vi "test-math-utils.vi"(8 "error in (no error)":errorcluster) -> (0 "error out":errorcluster, 3 "ALL TESTS PASSED":bool)   [LabVIEW 2019]
uses:
  <vilib>/Rock Robotics/WPI/ThirdParty/JAS_Junk/TrajLib/Trajectory_Library.lvlib
panel:
  out "Test 40":bool
  out "Test 39":bool
  out "Test 38":bool
  out "Test 37":bool
  out "Test 36":bool
  out "Test 35":bool
  out "Test 34":bool
  out "Test 33":bool
  out "Test 32":bool
  out "Test 31":bool
  out "Test 30":bool
  out "Test 29":bool
  out "Test 28":bool
  out "Test 27":bool
  out "Test 26":bool
  out "Test 25":bool
  out "mod 24":dbl
  out "Test 24":bool
  out "mod 23":dbl
  out "Test 23":bool
  out "mod 22":dbl
  out "Test 22":bool
  out "mod 21":dbl
  out "Test 21":bool
  out "mod 20":dbl
  out "Test 20":bool
  out "mod 19":dbl
  out "Test 19":bool
  out "mod 18":dbl
  out "mod 17":dbl
  out "mod 16":dbl
  out "Test 18":bool
  out "Test 17":bool
  out "Test 16":bool
  out "Test 15":bool
  out "Test 14":bool
  out "Test 13":bool
  out "Test 12":bool
  out "Test 11":bool
  out "Test 10":bool
  out "Test 9":bool
  out "Test 8":bool
  out "Test 7":bool
  out "Test 6":bool
  out "Test 5":bool
  out "Test 4":bool
  out "Test 3":bool
  out "Test 2":bool
  out "Test 1":bool
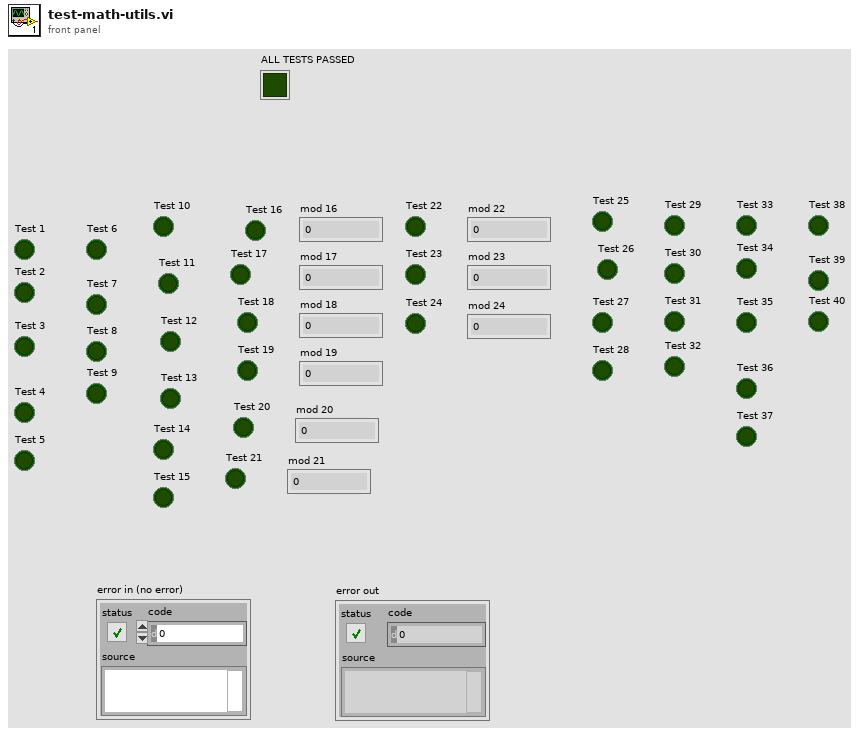
[diagram p1: front panel]
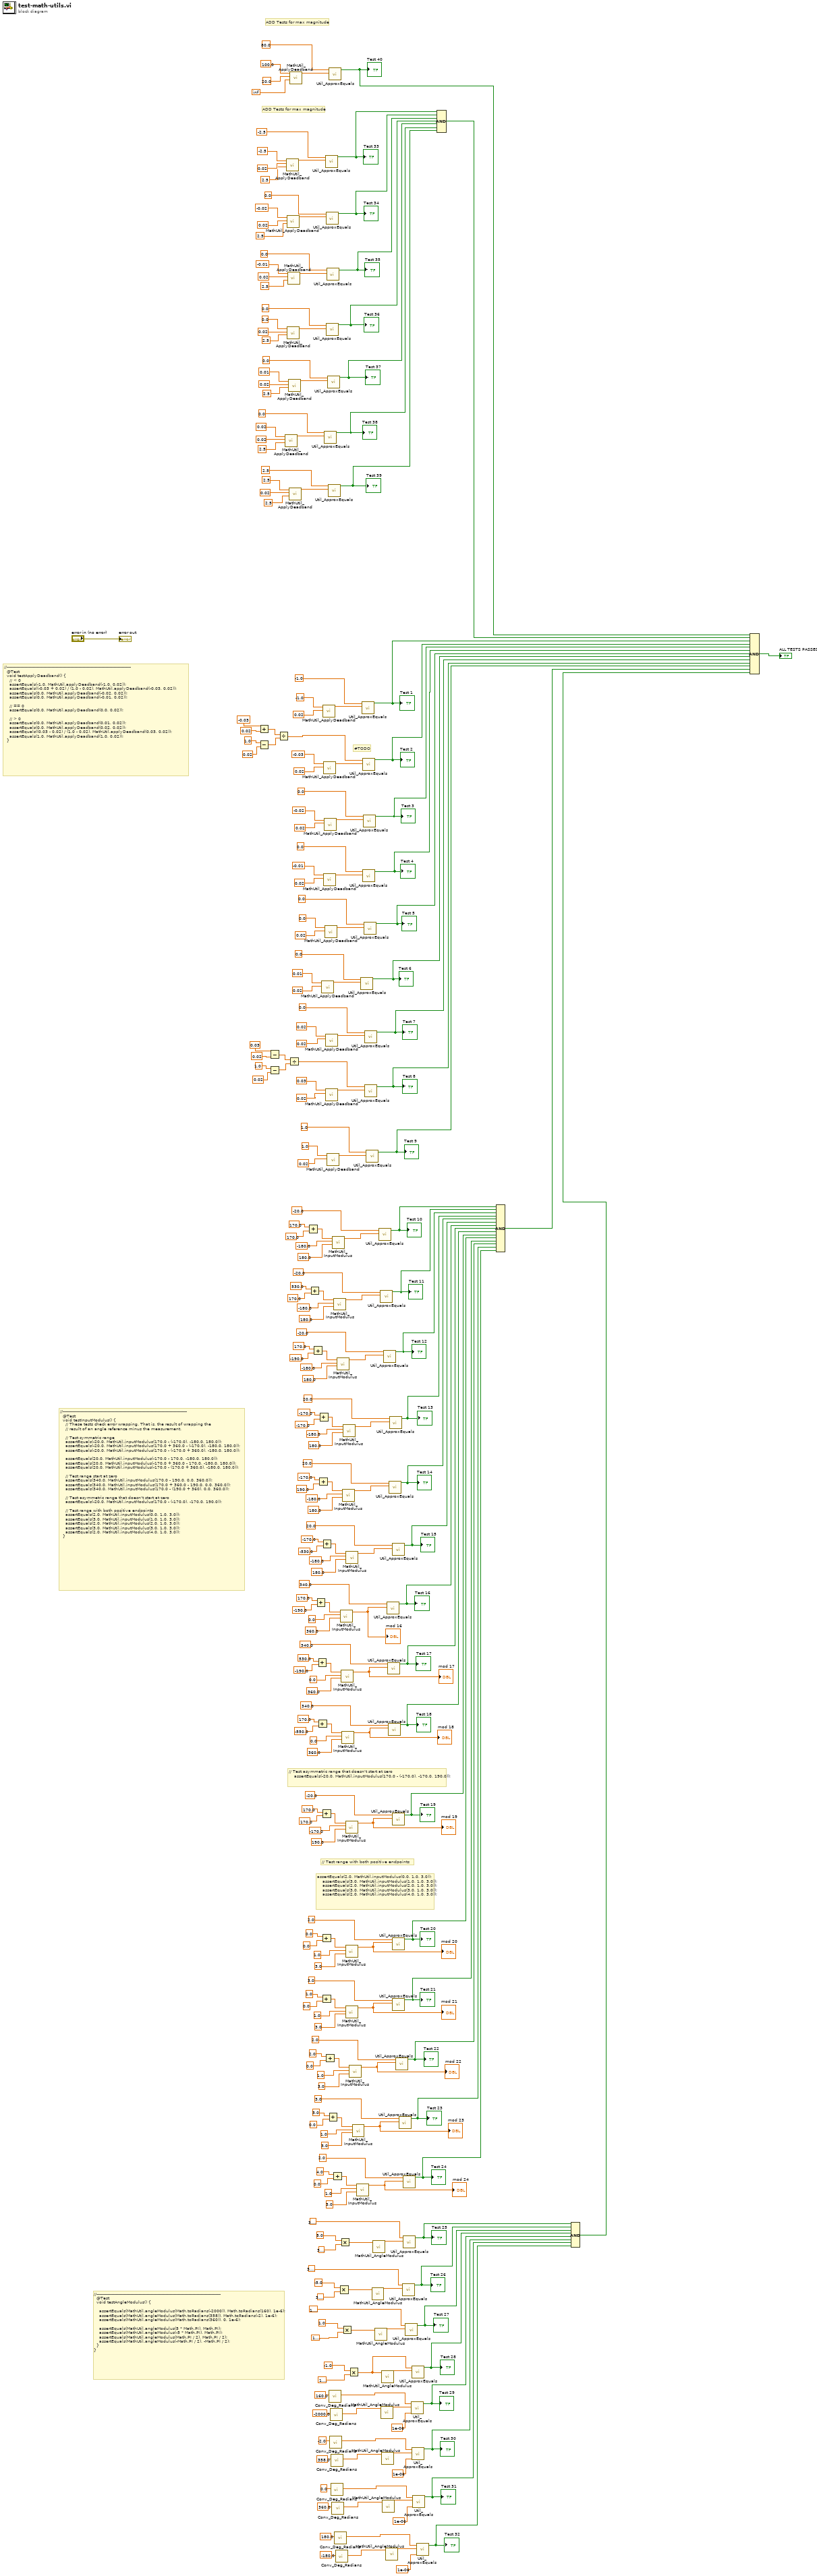
[diagram p0: block diagram]
diagram:
  # "ADD Tests for max magnitude"
  # "ADD Tests for max magnitude"
  # "assertEquals(2.0, MathUtil.inputModulus(0.0, 1.0, 3.0));\n    assertEquals(3.0, MathUtil.inputModulus(1.0, 1.0, 3.0));\n    assertEquals(2.0, MathUtil.inputModulus(2.0, 1.0, 3.0));\n    assertEquals(3.0, MathUtil.inputModulus(3.0, 1.0, 3.0));\n    assertEquals(2.0, MathUtil.inputModulus(4.0, 1.0, 3.0));"
  # "// Test range with both positive endpoints"
  # "// Test asymmetric range that doesn't start at zero\n    assertEquals(-20.0, MathUtil.inputModulus(170.0 - (-170.0), -170.0, 190.0));"
  # "#TODO"
  # "//--------------------------------------------------------------------------------------------\n  @Test\n  void testInputModulus() {\n    // These tests check error wrapping. That is, the result of wrapping the\n    // result of an angle reference minus the measurement.\n\n    // Test symmetric range\n    assertEquals(-20.0, MathUtil.inputModulus(170.0 - (-170.0), -180.0, 180.0));\n    assertEquals(-20.0, MathUtil.inputModulus(170.0 + 360.0 - (-170.0), -180.0, 180.0));\n    assertEquals(-20.0, MathUtil.inputModulus(170.0 - (-170.0 + 360.0), -180.0, 180.0));\n\n    assertEquals(20.0, MathUtil.inputModulus(-170.0 - 170.0, -180.0, 180.0));\n    assertEquals(20.0, MathUtil.inputModulus(-170.0 + 360.0 - 170.0, -180.0, 180.0));\n    assertEquals(20.0, MathUtil.inputModulus(-170.0 - (170.0 + 360.0), -180.0, 180.0));\n\n    // Test range start at zero\n    assertEquals(340.0, MathUtil.inputModulus(170.0 - 190.0, 0.0, 360.0));\n    assertEquals(340.0, MathUtil.inputModulus(170.0 + 360.0 - 190.0, 0.0, 360.0));\n    assertEquals(340.0, MathUtil.inputModulus(170.0 - (190.0 + 360), 0.0, 360.0));\n\n    // Test asymmetric range that doesn't start at zero\n    assertEquals(-20.0, MathUtil.inputModulus(170.0 - (-170.0), -170.0, 190.0));\n\n    // Test range with both positive endpoints\n    assertEquals(2.0, MathUtil.inputModulus(0.0, 1.0, 3.0));\n    assertEquals(3.0, MathUtil.inputModulus(1.0, 1.0, 3.0));\n    assertEquals(2.0, MathUtil.inputModulus(2.0, 1.0, 3.0));\n    assertEquals(3.0, MathUtil.inputModulus(3.0, 1.0, 3.0));\n    assertEquals(2.0, MathUtil.inputModulus(4.0, 1.0, 3.0));\n  }"
  # "//--------------------------------------------------------------------------------------------\n  @Test\n  void testApplyDeadband() {\n    // < 0\n    assertEquals(-1.0, MathUtil.applyDeadband(-1.0, 0.02));\n    assertEquals((-0.03 + 0.02) / (1.0 - 0.02), MathUtil.applyDeadband(-0.03, 0.02));\n    assertEquals(0.0, MathUtil.applyDeadband(-0.02, 0.02));\n    assertEquals(0.0, MathUtil.applyDeadband(-0.01, 0.02));\n\n    // == 0\n    assertEquals(0.0, MathUtil.applyDeadband(0.0, 0.02));\n\n    // > 0\n    assertEquals(0.0, MathUtil.applyDeadband(0.01, 0.02));\n    assertEquals(0.0, MathUtil.applyDeadband(0.02, 0.02));\n    assertEquals((0.03 - 0.02) / (1.0 - 0.02), MathUtil.applyDeadband(0.03, 0.02));\n    assertEquals(1.0, MathUtil.applyDeadband(1.0, 0.02));\n  }"
  # "//--------------------------------------------------------------------------------------------\n  @Test\n  void testAngleModulus() {\n\n    assertEquals(MathUtil.angleModulus(Math.toRadians(-2000)), Math.toRadians(160), 1e-6);\n    assertEquals(MathUtil.angleModulus(Math.toRadians(358)), Math.toRadians(-2), 1e-6);\n    assertEquals(MathUtil.angleModulus(Math.toRadians(360)), 0, 1e-6);\n\n    assertEquals(MathUtil.angleModulus(5 * Math.PI), Math.PI);\n    assertEquals(MathUtil.angleModulus(-5 * Math.PI), Math.PI);\n    assertEquals(MathUtil.angleModulus(Math.PI / 2), Math.PI / 2);\n    assertEquals(MathUtil.angleModulus(-Math.PI / 2), -Math.PI / 2);\n  }\n}"
  n1 = Add(x=-0.03, y=0.02) -> (x+y=w245:dbl)
  n2 = Subtract(x=1.0, y=0.02) -> (x-y=w244:dbl)
  n3 = Subtract(x=0.03, y=0.02) -> (x-y=w238:dbl)
  n4 = Subtract(x=1.0, y=0.02) -> (x-y=w237:dbl)
  n5 = Divide(x=w245, y=w244) -> (x/y=w239:dbl)
  n6 = call <vilib>:"MathUtil_ApplyDeadband.vi"("Max Magnitude"=2.5, "Deadband"=0.02, "Value"=0.02) -> ("Result"=w34:dbl)  [unwired: 8 in]
  n7 = call <vilib>:"MathUtil_ApplyDeadband.vi"("Max Magnitude"=2.5, "Deadband"=0.02, "Value"=-2.5) -> ("Result"=w48:dbl)  [unwired: 8 in]
  n8 = call <vilib>:"MathUtil_ApplyDeadband.vi"("Max Magnitude"=2.5, "Deadband"=0.02, "Value"=-0.02) -> ("Result"=w46:dbl)  [unwired: 8 in]
  n9 = call <vilib>:"MathUtil_ApplyDeadband.vi"("Max Magnitude"=2.5, "Deadband"=0.02, "Value"=0.0) -> ("Result"=w40:dbl)  [unwired: 8 in]
  n10 = call <vilib>:"MathUtil_ApplyDeadband.vi"("Max Magnitude"=2.5, "Deadband"=0.02, "Value"=-0.01) -> ("Result"=w43:dbl)  [unwired: 8 in]
  n11 = call <vilib>:"MathUtil_ApplyDeadband.vi"("Max Magnitude"=2.5, "Deadband"=0.02, "Value"=0.01) -> ("Result"=w37:dbl)  [unwired: 8 in]
  n12 = Divide(x=w238, y=w237) -> (x/y=w232:dbl)
  n13 = call <vilib>:"MathUtil_ApplyDeadband.vi"("Max Magnitude"=2.5, "Deadband"=0.02, "Value"=2.5) -> ("Result"=w31:dbl)  [unwired: 8 in]
  n14 = call <vilib>:"MathUtil_ApplyDeadband.vi"("Max Magnitude"=inf, "Deadband"=20.0, "Value"=100.0) -> ("Result"=w5:dbl)  [unwired: 8 in]
  n15 = Add(x=170.0, y=170.0) -> (x+y=w227:dbl)
  n16 = Add(x=530.0, y=170.0) -> (x+y=w220:dbl)
  n17 = Add(x=170.0, y=-190.0) -> (x+y=w213:dbl)
  n18 = Add(x=170.0, y=-190.0) -> (x+y=w185:dbl)
  n19 = Add(x=530.0, y=-190.0) -> (x+y=w178:dbl)
  n20 = Add(x=170.0, y=-550.0) -> (x+y=w171:dbl)
  n21 = Add(x=-170.0, y=190.0) -> (x+y=w199:dbl)
  n22 = Add(x=-170.0, y=-170.0) -> (x+y=w206:dbl)
  n23 = Add(x=170.0, y=170.0) -> (x+y=w164:dbl)
  n24 = Add(x=0.0, y=0.0) -> (x+y=w157:dbl)
  n25 = Add(x=1.0, y=0.0) -> (x+y=w150:dbl)
  n26 = Add(x=-170.0, y=-530.0) -> (x+y=w192:dbl)
  n27 = call <vilib>:"MathUtil_ApplyDeadband.vi"("Deadband"=0.02, "Value"=0.01) -> ("Result"=w265:dbl)  [unwired: 9 in]
  n28 = call <vilib>:"MathUtil_ApplyDeadband.vi"("Deadband"=0.02, "Value"=-1.0) -> ("Result"=w279:dbl)  [unwired: 9 in]
  n29 = call <vilib>:"MathUtil_ApplyDeadband.vi"("Deadband"=0.02, "Value"=-0.03) -> ("Result"=w277:dbl)  [unwired: 9 in]
  n30 = call <vilib>:"MathUtil_ApplyDeadband.vi"("Deadband"=0.02, "Value"=-0.01) -> ("Result"=w271:dbl)  [unwired: 9 in]
  n31 = call <vilib>:"MathUtil_ApplyDeadband.vi"("Deadband"=0.02, "Value"=-0.02) -> ("Result"=w274:dbl)  [unwired: 9 in]
  n32 = Add(x=2.0, y=0.0) -> (x+y=w143:dbl)
  n33 = call <vilib>:"Util_ApproxEquals.vi"("Value 2"=w34, "Value 1"=0.0) -> ("ApproxEquals"=w9:bool)  [unwired: 9 in]
  "Test 38" <- w9
  n34 = call <vilib>:"MathUtil_ApplyDeadband.vi"("Deadband"=0.02, "Value"=0.0) -> ("Result"=w268:dbl)  [unwired: 9 in]
  n35 = call <vilib>:"Util_ApproxEquals.vi"("Value 2"=w48, "Value 1"=-2.5) -> ("ApproxEquals"=w21:bool)  [unwired: 9 in]
  "Test 33" <- w21
  n36 = call <vilib>:"MathUtil_ApplyDeadband.vi"("Deadband"=0.02, "Value"=0.02) -> ("Result"=w262:dbl)  [unwired: 9 in]
  n37 = call <vilib>:"MathUtil_ApplyDeadband.vi"("Deadband"=0.02, "Value"=0.03) -> ("Result"=w260:dbl)  [unwired: 9 in]
  n38 = call <vilib>:"Util_ApproxEquals.vi"("Value 2"=w46, "Value 1"=0.0) -> ("ApproxEquals"=w20:bool)  [unwired: 9 in]
  "Test 34" <- w20
  n39 = call <vilib>:"Util_ApproxEquals.vi"("Value 2"=w40, "Value 1"=0.0) -> ("ApproxEquals"=w15:bool)  [unwired: 9 in]
  "Test 36" <- w15
  n40 = call <vilib>:"Util_ApproxEquals.vi"("Value 2"=w43, "Value 1"=0.0) -> ("ApproxEquals"=w19:bool)  [unwired: 9 in]
  "Test 35" <- w19
  n41 = call <vilib>:"MathUtil_ApplyDeadband.vi"("Deadband"=0.02, "Value"=1.0) -> ("Result"=w257:dbl)  [unwired: 9 in]
  n42 = Add(x=3.0, y=0.0) -> (x+y=w136:dbl)
  n43 = call <vilib>:"Util_ApproxEquals.vi"("Value 2"=w37, "Value 1"=0.0) -> ("ApproxEquals"=w12:bool)  [unwired: 9 in]
  "Test 37" <- w12
  n44 = call <vilib>:"Util_ApproxEquals.vi"("Value 2"=w31, "Value 1"=2.5) -> ("ApproxEquals"=w8:bool)  [unwired: 9 in]
  "Test 39" <- w8
  n45 = call <vilib>:"Util_ApproxEquals.vi"("Value 2"=w5, "Value 1"=80.0) -> ("ApproxEquals"=w1:bool)  [unwired: 9 in]
  "Test 40" <- w1
  n46 = call <vilib>:"Conv_Deg_Radians.vi"("Degress"=160.0) -> ("Radians"=w88:dbl)  [unwired: 10 in]
  n47 = call <vilib>:"Conv_Deg_Radians.vi"("Degress"=-2.0) -> ("Radians"=w82:dbl)  [unwired: 10 in]
  n48 = call <vilib>:"Conv_Deg_Radians.vi"("Degress"=-2000.0) -> ("Radians"=w87:dbl)  [unwired: 10 in]
  n49 = call <vilib>:"Conv_Deg_Radians.vi"("Degress"=0.0) -> ("Radians"=w76:dbl)  [unwired: 10 in]
  n50 = call <vilib>:"Conv_Deg_Radians.vi"("Degress"=358.0) -> ("Radians"=w81:dbl)  [unwired: 10 in]
  n51 = Add(x=4.0, y=0.0) -> (x+y=w129:dbl)
  n52 = call <vilib>:"Conv_Deg_Radians.vi"("Degress"=360.0) -> ("Radians"=w75:dbl)  [unwired: 10 in]
  n53 = call <vilib>:"MathUtil_InputModulus.vi"("Maximum_Input"=180.0, "Minimum_Input"=-180.0, "Input"=w227) -> ("modulus"=w231:dbl)  [unwired: 8 in]
  n54 = call <vilib>:"MathUtil_InputModulus.vi"("Maximum_Input"=180.0, "Minimum_Input"=-180.0, "Input"=w220) -> ("modulus"=w224:dbl)  [unwired: 8 in]
  n55 = call <vilib>:"Conv_Deg_Radians.vi"("Degress"=180.0) -> ("Radians"=w70:dbl)  [unwired: 10 in]
  n56 = call <vilib>:"Conv_Deg_Radians.vi"("Degress"=-180.0) -> ("Radians"=w69:dbl)  [unwired: 10 in]
  n57 = call <vilib>:"MathUtil_InputModulus.vi"("Maximum_Input"=180.0, "Minimum_Input"=-180.0, "Input"=w213) -> ("modulus"=w217:dbl)  [unwired: 8 in]
  n58 = Multiply(x=-5.0, y=3.141592653589793) -> (x*y=w103:dbl)
  n59 = Multiply(x=5.0, y=3.141592653589793) -> (x*y=w108:dbl)
  n60 = call <vilib>:"MathUtil_InputModulus.vi"("Maximum_Input"=360.0, "Minimum_Input"=0.0, "Input"=w185) -> ("modulus"=w189:dbl)  [unwired: 8 in]
  "mod 16" <- w189
  n61 = call <vilib>:"MathUtil_InputModulus.vi"("Maximum_Input"=360.0, "Minimum_Input"=0.0, "Input"=w178) -> ("modulus"=w182:dbl)  [unwired: 8 in]
  "mod 17" <- w182
  n62 = Multiply(x=1.0, y=1.5707963267948966) -> (x*y=w99:dbl)
  n63 = call <vilib>:"MathUtil_InputModulus.vi"("Maximum_Input"=360.0, "Minimum_Input"=0.0, "Input"=w171) -> ("modulus"=w175:dbl)  [unwired: 8 in]
  "mod 18" <- w175
  n64 = call <vilib>:"MathUtil_InputModulus.vi"("Maximum_Input"=180.0, "Minimum_Input"=-180.0, "Input"=w199) -> ("modulus"=w203:dbl)  [unwired: 8 in]
  n65 = call <vilib>:"MathUtil_InputModulus.vi"("Maximum_Input"=180.0, "Minimum_Input"=-180.0, "Input"=w206) -> ("modulus"=w210:dbl)  [unwired: 8 in]
  n66 = call <vilib>:"MathUtil_InputModulus.vi"("Maximum_Input"=190.0, "Minimum_Input"=-170.0, "Input"=w164) -> ("modulus"=w168:dbl)  [unwired: 8 in]
  "mod 19" <- w168
  n67 = call <vilib>:"MathUtil_InputModulus.vi"("Maximum_Input"=3.0, "Minimum_Input"=1.0, "Input"=w157) -> ("modulus"=w161:dbl)  [unwired: 8 in]
  "mod 20" <- w161
  n68 = call <vilib>:"MathUtil_InputModulus.vi"("Maximum_Input"=3.0, "Minimum_Input"=1.0, "Input"=w150) -> ("modulus"=w154:dbl)  [unwired: 8 in]
  "mod 21" <- w154
  n69 = call <vilib>:"MathUtil_InputModulus.vi"("Maximum_Input"=180.0, "Minimum_Input"=-180.0, "Input"=w192) -> ("modulus"=w196:dbl)  [unwired: 8 in]
  n70 = Multiply(x=-1.0, y=1.5707963267948966) -> (x*y=w92:dbl)
  n71 = call <vilib>:"MathUtil_InputModulus.vi"("Maximum_Input"=3.0, "Minimum_Input"=1.0, "Input"=w143) -> ("modulus"=w147:dbl)  [unwired: 8 in]
  "mod 22" <- w147
  n72 = call <vilib>:"MathUtil_InputModulus.vi"("Maximum_Input"=3.0, "Minimum_Input"=1.0, "Input"=w136) -> ("modulus"=w140:dbl)  [unwired: 8 in]
  "mod 23" <- w140
  n73 = call <vilib>:"MathUtil_InputModulus.vi"("Maximum_Input"=3.0, "Minimum_Input"=1.0, "Input"=w129) -> ("modulus"=w133:dbl)  [unwired: 8 in]
  "mod 24" <- w133
  n74 = call <vilib>:"Util_ApproxEquals.vi"("Value 2"=w265, "Value 1"=0.0) -> ("ApproxEquals"=w249:bool)  [unwired: 9 in]
  "Test 6" <- w249
  n75 = call <vilib>:"Util_ApproxEquals.vi"("Value 2"=w279, "Value 1"=-1.0) -> ("ApproxEquals"=w254:bool)  [unwired: 9 in]
  "Test 1" <- w254
  n76 = call <vilib>:"Util_ApproxEquals.vi"("Value 2"=w277, "Value 1"=w239) -> ("ApproxEquals"=w253:bool)  [unwired: 9 in]
  "Test 2" <- w253
  n77 = call <vilib>:"Util_ApproxEquals.vi"("Value 2"=w271, "Value 1"=0.0) -> ("ApproxEquals"=w251:bool)  [unwired: 9 in]
  "Test 4" <- w251
  n78 = call <vilib>:"Util_ApproxEquals.vi"("Value 2"=w274, "Value 1"=0.0) -> ("ApproxEquals"=w252:bool)  [unwired: 9 in]
  "Test 3" <- w252
  n79 = call <vilib>:"Util_ApproxEquals.vi"("Value 2"=w268, "Value 1"=0.0) -> ("ApproxEquals"=w250:bool)  [unwired: 9 in]
  "Test 5" <- w250
  n80 = call <vilib>:"Util_ApproxEquals.vi"("Value 2"=w262, "Value 1"=0.0) -> ("ApproxEquals"=w248:bool)  [unwired: 9 in]
  "Test 7" <- w248
  n81 = call <vilib>:"Util_ApproxEquals.vi"("Value 2"=w260, "Value 1"=w232) -> ("ApproxEquals"=w247:bool)  [unwired: 9 in]
  "Test 8" <- w247
  n82 = call <vilib>:"Util_ApproxEquals.vi"("Value 2"=w257, "Value 1"=1.0) -> ("ApproxEquals"=w246:bool)  [unwired: 9 in]
  "Test 9" <- w246
  n83 = call <vilib>:"MathUtil_AngleModulus.vi"("InputAngle"=w103) -> ("ModulsAngle"=w105:dbl)  [unwired: 10 in]
  n84 = call <vilib>:"MathUtil_AngleModulus.vi"("InputAngle"=w108) -> ("ModulsAngle"=w110:dbl)  [unwired: 10 in]
  n85 = call <vilib>:"MathUtil_AngleModulus.vi"("InputAngle"=w99) -> ("ModulsAngle"=w100:dbl)  [unwired: 10 in]
  n86 = call <vilib>:"Util_ApproxEquals.vi"("Value 2"=w231, "Value 1"=-20.0) -> ("ApproxEquals"=w126:bool)  [unwired: 9 in]
  "Test 10" <- w126
  n87 = call <vilib>:"Util_ApproxEquals.vi"("Value 2"=w224, "Value 1"=-20.0) -> ("ApproxEquals"=w125:bool)  [unwired: 9 in]
  "Test 11" <- w125
  n88 = call <vilib>:"MathUtil_AngleModulus.vi"("InputAngle"=w87) -> ("ModulsAngle"=w91:dbl)  [unwired: 10 in]
  n89 = call <vilib>:"MathUtil_AngleModulus.vi"("InputAngle"=w92) -> ("ModulsAngle"=w95:dbl)  [unwired: 10 in]
  n90 = call <vilib>:"MathUtil_AngleModulus.vi"("InputAngle"=w81) -> ("ModulsAngle"=w85:dbl)  [unwired: 10 in]
  n91 = call <vilib>:"MathUtil_AngleModulus.vi"("InputAngle"=w75) -> ("ModulsAngle"=w79:dbl)  [unwired: 10 in]
  n92 = call <vilib>:"Util_ApproxEquals.vi"("Value 2"=w217, "Value 1"=-20.0) -> ("ApproxEquals"=w124:bool)  [unwired: 9 in]
  "Test 12" <- w124
  n93 = call <vilib>:"MathUtil_AngleModulus.vi"("InputAngle"=w69) -> ("ModulsAngle"=w73:dbl)  [unwired: 10 in]
  n94 = call <vilib>:"Util_ApproxEquals.vi"("Value 2"=w189, "Value 1"=340.0) -> ("ApproxEquals"=w120:bool)  [unwired: 9 in]
  "Test 16" <- w120
  n95 = call <vilib>:"Util_ApproxEquals.vi"("Value 2"=w182, "Value 1"=340.0) -> ("ApproxEquals"=w119:bool)  [unwired: 9 in]
  "Test 17" <- w119
  n96 = call <vilib>:"Util_ApproxEquals.vi"("Value 2"=w175, "Value 1"=340.0) -> ("ApproxEquals"=w118:bool)  [unwired: 9 in]
  "Test 18" <- w118
  n97 = call <vilib>:"Util_ApproxEquals.vi"("Value 2"=w203, "Value 1"=20.0) -> ("ApproxEquals"=w122:bool)  [unwired: 9 in]
  "Test 14" <- w122
  n98 = call <vilib>:"Util_ApproxEquals.vi"("Value 2"=w210, "Value 1"=20.0) -> ("ApproxEquals"=w123:bool)  [unwired: 9 in]
  "Test 13" <- w123
  n99 = call <vilib>:"Util_ApproxEquals.vi"("Value 2"=w168, "Value 1"=-20.0) -> ("ApproxEquals"=w117:bool)  [unwired: 9 in]
  "Test 19" <- w117
  n100 = call <vilib>:"Util_ApproxEquals.vi"("Value 2"=w161, "Value 1"=2.0) -> ("ApproxEquals"=w116:bool)  [unwired: 9 in]
  "Test 20" <- w116
  n101 = call <vilib>:"Util_ApproxEquals.vi"("Value 2"=w154, "Value 1"=3.0) -> ("ApproxEquals"=w115:bool)  [unwired: 9 in]
  "Test 21" <- w115
  n102 = call <vilib>:"Util_ApproxEquals.vi"("Value 2"=w196, "Value 1"=20.0) -> ("ApproxEquals"=w121:bool)  [unwired: 9 in]
  "Test 15" <- w121
  n103 = call <vilib>:"Util_ApproxEquals.vi"("Value 2"=w147, "Value 1"=2.0) -> ("ApproxEquals"=w114:bool)  [unwired: 9 in]
  "Test 22" <- w114
  n104 = call <vilib>:"Util_ApproxEquals.vi"("Value 2"=w140, "Value 1"=3.0) -> ("ApproxEquals"=w113:bool)  [unwired: 9 in]
  "Test 23" <- w113
  n105 = call <vilib>:"Util_ApproxEquals.vi"("Value 2"=w105, "Value 1"=3.141592653589793) -> ("ApproxEquals"=w66:bool)  [unwired: 9 in]
  "Test 26" <- w66
  n106 = call <vilib>:"Util_ApproxEquals.vi"("Value 2"=w133, "Value 1"=2.0) -> ("ApproxEquals"=w112:bool)  [unwired: 9 in]
  "Test 24" <- w112
  n107 = call <vilib>:"Util_ApproxEquals.vi"("Value 2"=w110, "Value 1"=3.141592653589793) -> ("ApproxEquals"=w67:bool)  [unwired: 9 in]
  "Test 25" <- w67
  n108 = call <vilib>:"Util_ApproxEquals.vi"("Value 2"=w100, "Value 1"=1.5707963267948966) -> ("ApproxEquals"=w65:bool)  [unwired: 9 in]
  "Test 27" <- w65
  n109 = call <vilib>:"Util_ApproxEquals.vi"("Tolerance"=1e-06, "Value 2"=w91, "Value 1"=w88) -> ("ApproxEquals"=w63:bool)  [unwired: 8 in]
  "Test 29" <- w63
  n110 = call <vilib>:"Util_ApproxEquals.vi"("Value 2"=w95, "Value 1"=w92) -> ("ApproxEquals"=w64:bool)  [unwired: 9 in]
  "Test 28" <- w64
  n111 = call <vilib>:"Util_ApproxEquals.vi"("Tolerance"=1e-06, "Value 2"=w85, "Value 1"=w82) -> ("ApproxEquals"=w62:bool)  [unwired: 8 in]
  "Test 30" <- w62
  n112 = call <vilib>:"Util_ApproxEquals.vi"("Tolerance"=1e-06, "Value 2"=w79, "Value 1"=w76) -> ("ApproxEquals"=w61:bool)  [unwired: 8 in]
  "Test 31" <- w61
  n113 = call <vilib>:"Util_ApproxEquals.vi"("Tolerance"=1e-06, "Value 2"=w73, "Value 1"=w70) -> ("ApproxEquals"=w60:bool)  [unwired: 8 in]
  "Test 32" <- w60
  n114 = Compound Arithmetic op=AND(w21, w20, w19, w15, w12, w9, w8) -> (w7:bool)
  n115 = Compound Arithmetic op=AND(w126, w125, w124, w123, w122, w121, w120, w119, w118, w117, w116, w115, w114, w113, w112) -> (w111:bool)
  n116 = Compound Arithmetic op=AND(w67, w66, w65, w64, w63, w62, w61, w60) -> (w59:bool)
  n117 = Compound Arithmetic op=AND(w1, w7, w254, w253, w252, w251, w250, w249, w248, w247, w246, w111, w59) -> (→"ALL TESTS PASSED":bool)
  "error out" <- "error in (no error)"
